vi "UHR-Fleezers Control (host) -TL FB Corrected Ronen semipassive - stepping.vi"(0 "Tab Control":T5(tab)=enum."Trap Control (RF)") -> ()   [LabVIEW 2013] (continued)
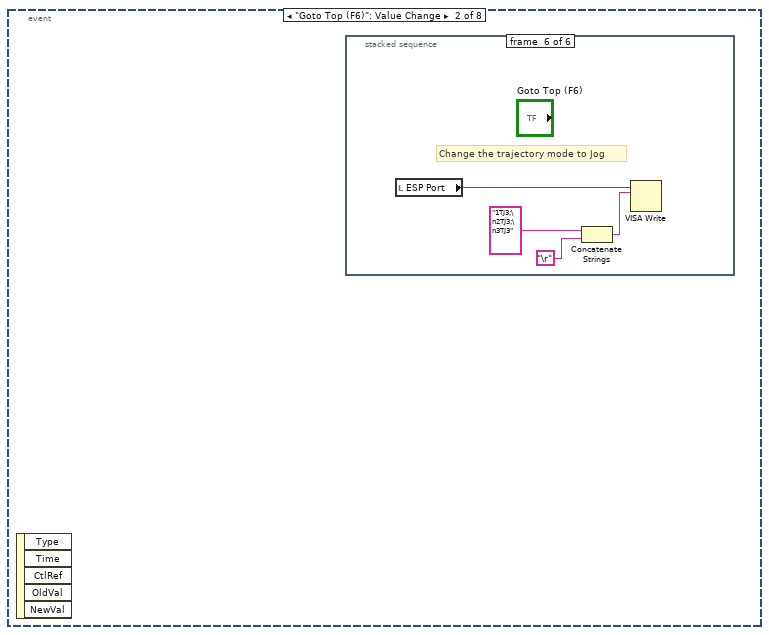
[diagram p4: hidden frame]
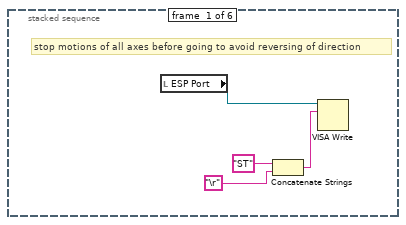
[diagram p5: hidden frame]
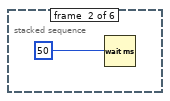
[diagram p6: hidden frame]
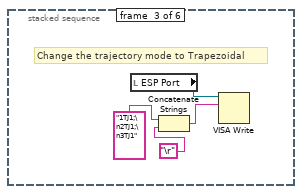
[diagram p7: hidden frame]
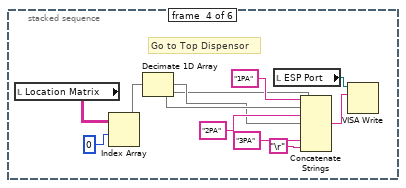
[diagram p8: hidden frame]
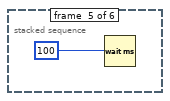
[diagram p9: hidden frame]
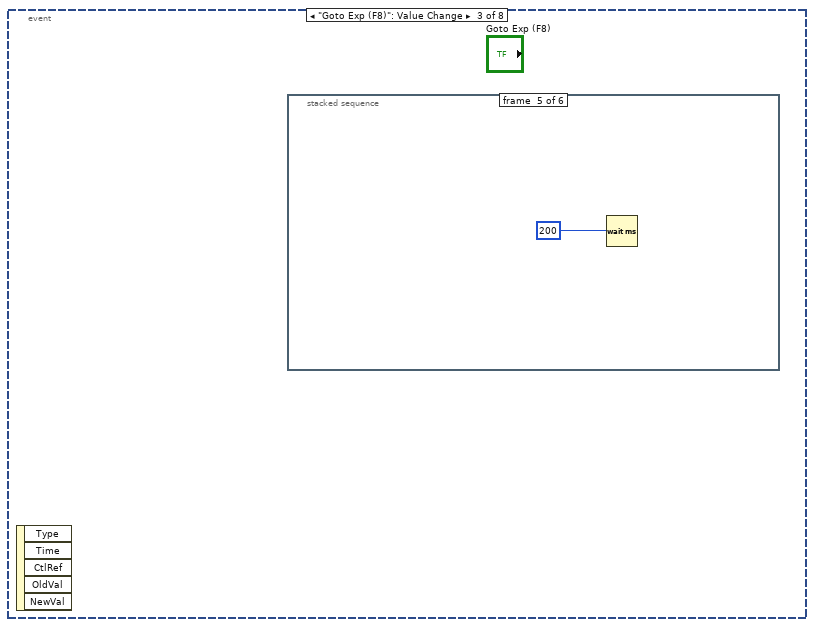
[diagram p10: hidden frame]
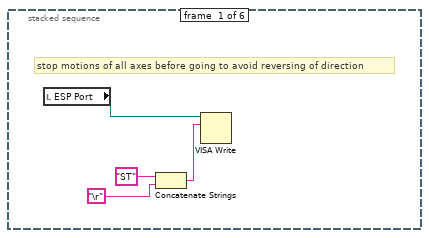
[diagram p11: hidden frame]
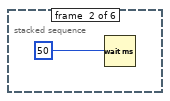
[diagram p12: hidden frame]
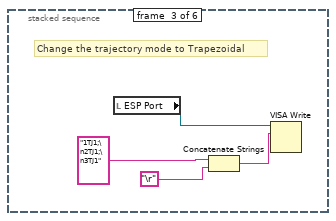
[diagram p13: hidden frame]
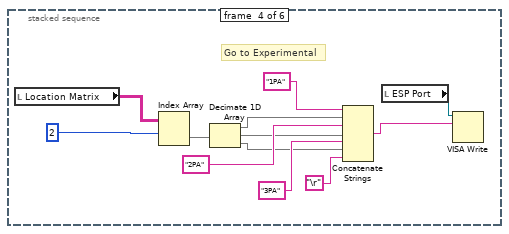
[diagram p14: hidden frame]
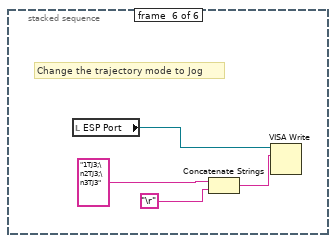
[diagram p15: hidden frame]
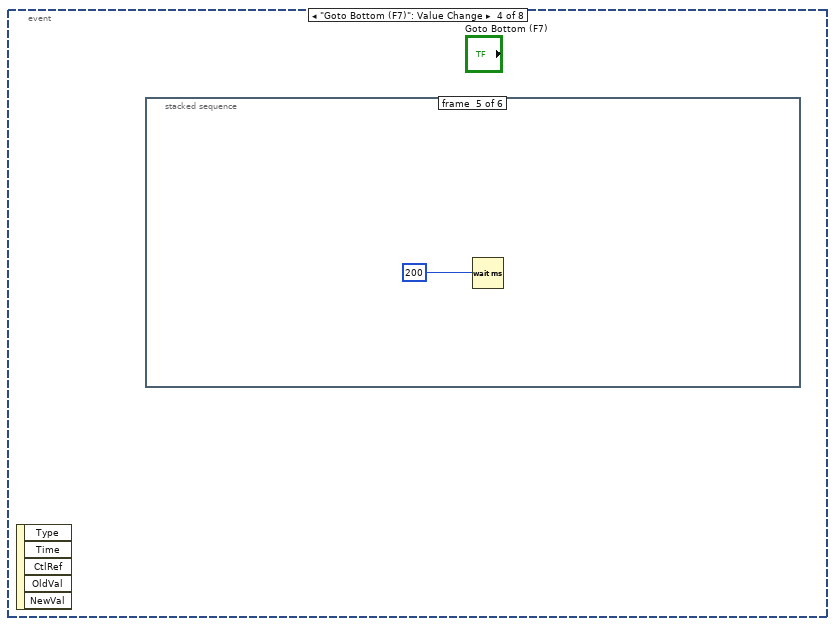
[diagram p16: hidden frame]
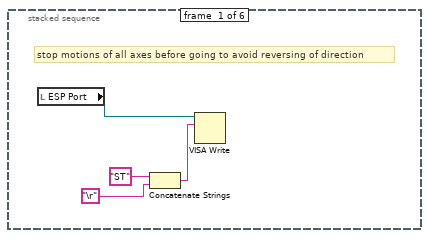
[diagram p17: hidden frame]
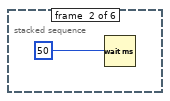
[diagram p18: hidden frame]
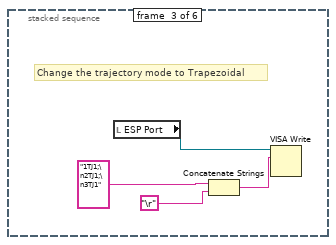
[diagram p19: hidden frame]
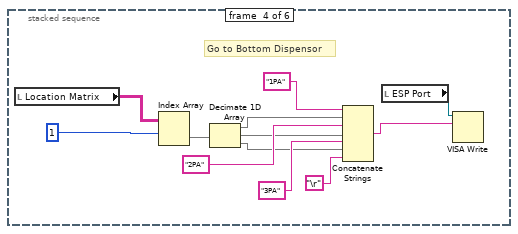
[diagram p20: hidden frame]
                n2311 = call-poly <vilib>:"Mean.vi"("X"=w3787) -> ("mean"=w3780:dbl)  [unwired: 1 out]
                n2312 = Subtract(x=w3781, y=w3780) -> (x-y=w3771:dbl)
                "Delta Fl. 2" <- w3771
                n2313 = Subtract(x=w3806, y=w3805) -> (x-y=w3803:dbl)
                "Delta Fl. 1" <- w3803
                n2314 = Initialize Array(w3803, 1 ("dimension size")) -> (w3800:dbl[])
                n2315 = Initialize Array(w3771, 1 ("dimension size")) -> (w3777:dbl[])
                n2316 = feedback #29(w3800) -> (w3801:dbl[])
                n2317 = Build Array (concatenate)(w3801, w3800) -> (w3799:dbl[])
                n2318 = feedback #30(w3777) -> (w3778:dbl[])
                n2319 = Build Array (concatenate)(w3778, w3777) -> (w3776:dbl[])
                n2320 = Select(t=w3800, s=w3772, f=w3799) -> (s? t:f=w3775:dbl[])
                n2321 = feedback-in #29(w3775) -> ()
                n2322 = Select(t=w3777, s=w3772, f=w3776) -> (s? t:f=w3774:dbl[])
                n2323 = feedback-in #30(w3774) -> ()
                n2324 = Build Array(w3775, w3774) -> (→"Save APD Deriv":dbl[][])
              }
            }
            "Progress" <- w3748
            "Progress 2" <- w3748
          }
        }
      }
    }
    n2325 = Bundle By Name(cluster=w2398, "Green FB Ch 0"=w2397, "Green FB Ch 1"=w2396) -> (w2380:T49)
    "Green FB Signals (V)" <- w2380
    n2326 = Unbundle By Name(w2380) -> ("Green FB Ch 2"=→"Green FB Plot":dbl)
    n2327 = local read "wait to reset values"() -> (w2466:bool)
    n2328 = Not(x=w2463) -> (.not. x?=w2467:bool)
    n2329 = And(x=w2467, y=w2466) -> (x .and. y?=w2468:bool)
    n2330 = case "Part of MCL raster scanning: returns to initial positions after scan done" shown="False" w2468 {
      tunnel: w2471 -> [w3300 w3307]
      tunnel: [w3300 w3306] -> w2470
      tunnel: w2465 -> [w3299 w3305]
      tunnel: [w3299 w3304] -> w2464
      frame False {
      }
      frame True {
        w3315 = 10.0 ("y")
        w3314 = 32767.0 ("y")
        # "to return scan values\nafter a synchronous \nAOM scan"
        n2331 = local read "AO2"() -> (w3308:dbl)
        n2332 = local read "AO1"() -> (w3309:dbl)
        n2333 = local write "wait to reset values"(FALSE ("wait to reset values")) -> ()
        n2334 = Multiply(x=w3309, y=w3314) -> (x*y=w3311:dbl)
        n2335 = Multiply(x=w3308, y=w3314) -> (x*y=w3313:dbl)
        n2336 = Divide(x=w3311, y=w3315) -> (x/y=w3310:dbl)
        n2337 = Divide(x=w3313, y=w3315) -> (x/y=w3312:dbl)
        n2338 = To Word Integer(number=w3310) -> (16bit integer=w3316:i16)
        n2339 = To Word Integer(number=w3312) -> (16bit integer=w3317:i16)
        n2340 = local read "Total Counts (ticks)"() -> (w3301:u32)
        n2341 = xnode "Read/Write Control"("FPGA VI Reference In"=w3307, "error in"=w3305, "AO1"=w3316, "AO2"=w3317, "MCL count"=w3301) -> ("FPGA VI Reference Out"=w3306:T20, "error out"=w3304:errorcluster)
        n2342 = local read "Scan Range (V)\n(of steps)"() -> (w3302:dbl)
        n2343 = property on="Scan Range (V)\n(of steps)" class="DigNum (strict)"("Val(Sgnl)"=w3302) -> ()  [unwired: 2 in, 2 out]
      }
    }
    n2344 = node-c288() -> ()  [unwired: 2 out]
  }
  n2345 = node-c288(3 ("Processor")) -> (w94:T25)  [unwired: 3 out]
  n2346 = timed-loop "Oscillate AOD (debugging)" {
    tunnel: w44 -> [w3876]
    tunnel: [w3875] -> w56
    timing: w94 -> [_]
    timing-out: [_] -> w93
    stop <- w3875 stop-if-true
    n2347 = node-c288() -> ()  [unwired: 2 out]
    n2348 = event shown="[0] \"Oscillate Set 2\", \"Fish for Tether\": Value Change" {
      selector: _ -> [_ _ _]
      dyn-events: _ -> [_ _ _]
      timeout: _ -> [_ _ _]
      tunnel: w3876 -> [w3883 _ _]
      tunnel: [FALSE ("Stop All") _ w4151] -> w3875
      event "Oscillate Set 2", "Fish for Tether": Value Change {
        n2349 = event-data() -> ()  [unwired: 6 out]
        n2350 = local read "Oscillate Set 2"() -> (w3882:bool)
        n2351 = Or(x=w3882, y="Fish for Tether") -> (x .or. y?=w3880:bool)
        n2352 = case shown="True" w3880 {
          tunnel: w3883 -> [_ w3886]
          tunnel: "Fish for Tether" -> [_ w3885]
          frame False {
          }
          frame True {
            n2353 = case shown="True" w3885 {
              frame False {
              }
              frame True {
                n2354 = local write "Scan axis 2"(TRUE) -> ()
                n2355 = local write "Tether"(FALSE ("Tether")) -> ()
              }
            }
            n2356 = node-c288("Period") -> (w3888:T25)  [unwired: 3 out]
            n2357 = timed-loop "Oscillate AOD" {
              timing: w3888 -> [_]
              timing-out: [_] -> w3887
              tunnel: w3886 -> [w3898]
              tunnel: w3885 -> [w3897]
              i -> [w3900]
              stop <- w3896 stop-if-true
              n2358 = node-c288() -> (w3899:i64)  [unwired: 1 out]
              n2359 = flat-sequence {
                tunnel: w3900 -> [w3926]
                tunnel: w3899 -> [w3925]
                tunnel: w3898 -> [w3909]
                tunnel: w3897 -> [w3911]
                tunnel: [w3911] -> w3895
                tunnel: [w3910] -> w3894
                tunnel: [w3908] -> w3893
                tunnel: [w3905] -> w3891
                tunnel: w3895 -> [w3962]
                tunnel: w3894 -> [w3960]
                tunnel: w3893 -> [w3959]
                tunnel: [w3958] -> w3892
                tunnel: w3891 -> [w3957]
                tunnel: [w4026] -> w3896
                tunnel: w3892 -> [w4024]
                frame #0 {
                  n2360 = Divide(x=w3925, y=i64 1000) -> (x/y=w3920:dbl)
                  n2361 = Multiply(x=w3920, y=w3926) -> (x*y=w3922:dbl)
                  n2362 = Multiply(x="Osc. freq. (Hz)", y=6.283185307179586) -> (x*y=w3923:dbl)
                  n2363 = Multiply(x=w3923, y=w3922) -> (x*y=w3907:dbl)
                  n2364 = local read "BD 1 Frequency 2 (MHz)"() -> (w3904:dbl)
                  n2365 = local read "BD 1 Frequency 1 (MHz)"() -> (w3901:dbl)
                  n2366 = case shown="True" w3911 {
                    tunnel: w3907 -> [w3932 w3939]
                    tunnel: w3904 -> [_ w3949]
                    tunnel: [w3929 w3933] -> w3912
                    tunnel: [FALSE w3942] -> w3908
                    tunnel: [0.0 w3935] -> w3905
                    tunnel: w3901 -> [_ w3934]
                    frame False {
                      n2367 = Sine(x=w3932) -> (sin(x)=w3930:dbl)
                      n2368 = Multiply(x=w3930, y="Osc. amp. (MHz)") -> (x*y=w3929:dbl)
                    }
                    frame True {
                      n2369 = Cosine(x=w3939) -> (cos(x)=w3952:dbl)
                      n2370 = Subtract(x=w3949, y=w3934) -> (x-y=w3948:dbl)
                      n2371 = Decrement(x=w3952) -> (x-1=w3951:dbl)
                      n2372 = Subtract(x=w3948, y="Closest Delta (MHz)") -> (x-y=w3945:dbl)
                      n2373 = Divide(x=w3951, y=2.0) -> (x/y=w3946:dbl)
                      n2374 = Multiply(x=w3946, y=w3945) -> (x*y=w3933:dbl)
                      n2375 = local read "Vec Mean of T1 T2"() -> (w3941:dbl[])
                      n2376 = Greater?(x=w3941, y="Stop F (pN)") -> (0:w3943:bool[])
                      n2377 = Or Array Elements(Boolean array=w3943) -> (logical OR=w3942:bool)
                      n2378 = Divide(x=w3939, y=6.283185307179586) -> (x/y=w3938:dbl)
                      n2379 = Round Toward +Infinity(x=w3938) -> (ceil(x): smallest int >= x=w3935:dbl)
                      "Attempts" <- w3935
                      n2380 = Greater?(x=w3935, y="Attempt Limit") -> (0:w3937:bool)
                      n2381 = case shown="True" w3937 {
                        frame False {
                        }
                        frame True {
                          n2382 = local write "Fish for Tether"(FALSE ("Fish for Tether")) -> ()
                          n2383 = call <vilib>:"Beep.vi"() -> ()  [unwired: 3 in, 9 out]
                          n2384 = local read "Messages"() -> (w3954:string)
                          n2385 = call "Update messages.vi"("Message to add"="Tether fishing timeout." ("Messages"), "Old message string"=w3954) -> ("New message string"=→"Messages":string)
                        }
                      }
                    }
                  }
                  n2386 = local read "Y RF Frequency Limits (MHz)"() -> (w3913:T17)
                  n2387 = local read "X RF Frequency Limits (MHz)"() -> (w3914:T17)
                  n2388 = local read "BD 1 Frequency 3 (MHz)"() -> (w3919:dbl)
                  n2389 = local read "BD 2 Frequency 2 (MHz)"() -> (w3903:dbl)
                  n2390 = Select(t=w3904, s="Scan axis 2", f=w3903) -> (s? t:f=w3915:dbl)
                  n2391 = Add(x=w3912, y=w3915) -> (x+y=w3910:dbl)
                  n2392 = Select(t=w3910, s="Scan axis 2", f=w3904) -> (s? t:f=w3902:dbl)
                  n2393 = Select(t=w3903, s="Scan axis 2", f=w3910) -> (s? t:f=w3917:dbl)
                  n2394 = local read "BD 2 Frequency 3 (MHz)"() -> (w3918:dbl)
                  n2395 = call "set RF board frequency - interlace.vi"("Board 2 Frequency Limits"=w3913, "Board 1 Frequency Limits"=w3914, "FPGA VI Reference In"=w3909, "Board 2 Frequency 3 (MHz)"=w3918, "Board 1 Frequency 3 (MHz)"=w3919, "Board 2 Frequency 2 (MHz)"=w3903, "Board 2 Frequency 1 (MHz)"=w3917, "Board 1 Frequency 2 (MHz)"=w3902, "Board 1 Frequency 1  (MHz)"=w3901) -> ()  [unwired: 1 in, 2 out]
                }
                frame #1 {
                  n2396 = And(x=w3962, y=w3959) -> (x .and. y?=w3961:bool)
                  n2397 = case "Only if were fishing and now formed tether" shown="True" w3961 {
                    tunnel: w3960 -> [w3964 w3976]
                    tunnel: [w3963 w3975] -> w3958
                    tunnel: w3957 -> [_ w3971]
                    frame False {
                      n2398 = local read "Fish for Tether"() -> (w3963:bool)
                      n2399 = case shown="True" w3963 {
                        tunnel: w3964 -> [_ _]
                        frame False {
                        }
                        frame True {
                        }
                      }
                    }
                    frame True {
                      w3975 = FALSE ("Fish for Tether")
                      n2400 = call <vilib>:"Beep.vi"() -> ()  [unwired: 3 in, 9 out]
                      n2401 = Number To Decimal String(number=w3971, width (-)=i16 1) -> (decimal integer string=w3969:string)
                      n2402 = case shown="\"2\", \"3\", \"4\", \"5\", \"6\"" "Then..." {
                        selector: "Then..." -> [_ w3979]
                        tunnel: w3976 -> [w3978 _]
                        frame "1", Default {
                          # "do nothing"
                          n2403 = property on="BD 1 Frequency 1 (MHz)" class="DigNum (strict)"("Val(Sgnl)"=w3978) -> ()  [unwired: 2 in, 2 out]
                        }
                        frame "2", "3", "4", "5", "6" {
                          n2404 = flat-sequence {
                            tunnel: w3979 -> [w3981]
                            frame #0 {
                              n2405 = property on="Trap Delta (MHz)" class="DigNum (strict)"("Val(Sgnl)"="Move to Delta 1 (MHz)") -> ()  [unwired: 2 in, 2 out]
                            }
                            frame #1 {
                              n2406 = case shown="\"5\", \"6\"" w3981 {
                                selector: w3981 -> [w3984 w3994 _]
                                frame "3", "4" {
                                n2407 = flat-sequence {
                                tunnel: w3984 -> [w3985]
                                tunnel: [w3985] -> w3982
                                tunnel: [w3987] -> w3983
                                tunnel: w3982 -> [w3987]
                                tunnel: w3983 -> [w3991]
                                frame #0 {
                                n2408 = property on="Green Laser ON/Interlacing" class="Bool (strict)"("Val(Sgnl)"=TRUE ("Value (Signaling)")) -> ()  [unwired: 2 in, 2 out]
                                }
                                frame #1 {
                                n2409 = Multiply(x="Wait Before Save (s)", y=u32 1000 ("x")) -> (x*y=w3989:u32)
                                n2410 = Wait (ms)(milliseconds to wait=w3989) -> ()  [unwired: 1 out]
                                }
                                frame #2 {
                                n2411 = property on="Start Saving" class="Bool (strict)"("Value"=TRUE ("Start Saving")) -> ()  [unwired: 2 in, 2 out]
                                n2412 = case shown="Default" w3991 {
                                frame Default {
                                }
                                frame "4" {
                                n2413 = property on="Fl. Triggered..." class="Bool (strict)"("Val(Sgnl)"=TRUE ("Value (Signaling)")) -> ()  [unwired: 2 in, 2 out]
                                }
                                }
                                }
                                }
                                }
                                frame "5", "6" {
                                n2414 = stacked-sequence {
                                tunnel: w3994 -> [_ _ _ _ _ _ _ _ w4011 _ _]
                                frame #0 {
                                n2415 = Replace Array Subset(array=u32[] [0] ("Index Values"), new element="Raster Set Upon Tether", index=0) -> (w3995:u32[])
                                n2416 = property on="Saved AOD Raster Scan Parameter Sets" class="Arr (strict)"("Index Values"=w3995) -> ()  [unwired: 2 in, 2 out]
                                }
                                frame #1 {
                                n2417 = Wait (ms)(milliseconds to wait=u32 500) -> ()  [unwired: 1 out]
                                }
                                frame #2 {
                                n2418 = property on="Load parameters" class="Bool (strict)"("Val(Sgnl)"=TRUE ("Value (Signaling)")) -> ()  [unwired: 2 in, 2 out]
                                }
                                frame #3 {
                                n2419 = Wait (ms)(milliseconds to wait=u32 500) -> ()  [unwired: 1 out]
                                }
                                frame #4 {
                                n2420 = property on="Trap Raster Scan" class="Bool (strict)"("Val(Sgnl)"=TRUE ("Value (Signaling)")) -> ()  [unwired: 2 in, 2 out]
                                }
                                frame #5 {
                                n2421 = Wait (ms)(milliseconds to wait=u32 2000) -> ()  [unwired: 1 out]
                                }
                                frame #6 {
                                n2422 = while {
                                stop <- w4006 stop-if-true
                                n2423 = local read "Raster Scanning..."() -> (w4005:bool)
                                n2424 = local read "Saving..."() -> (w4008:bool)
                                n2425 = Wait (ms)(milliseconds to wait=u32 100) -> ()  [unwired: 1 out]
                                n2426 = Not(x=w4008) -> (.not. x?=w4007:bool)
                                n2427 = Not(x=w4005) -> (.not. x?=w4004:bool)
                                n2428 = And(x=w4007, y=w4004) -> (x .and. y?=w4006:bool)
                                }
                                }
                                frame #7 {
                                n2429 = property on="Trap Delta (MHz)" class="DigNum (strict)"("Val(Sgnl)"="Move to Delta 2 (MHz)") -> ()  [unwired: 2 in, 2 out]
                                }
                                frame #8 {
                                n2430 = local read "Tether"() -> (w4012:bool)
                                n2431 = case shown="True" w4012 {
                                tunnel: w4011 -> [_ w4013]
                                frame False {
                                }
                                frame True {
                                n2432 = flat-sequence {
                                tunnel: w4013 -> [w4015]
                                frame #0 {
                                n2433 = Wait (ms)(milliseconds to wait=u32 500) -> ()  [unwired: 1 out]
                                }
                                frame #1 {
                                n2434 = case shown="\"6\"" w4015 {
                                frame Default {
                                }
                                frame "6" {
                                n2435 = property on="Green Laser ON/Interlacing" class="Bool (strict)"("Val(Sgnl)"=TRUE ("Green Laser ON/Interlacing")) -> ()  [unwired: 2 in, 2 out]
                                }
                                }
                                }
                                frame #2 {
                                n2436 = Wait (ms)(milliseconds to wait=u32 500) -> ()  [unwired: 1 out]
                                }
                                frame #3 {
                                n2437 = local write "Start Saving"("Save at end (5, 6)") -> ()
                                }
                                }
                                }
                                }
                                }
                                frame #9 {
                                n2438 = local read "Bead Sep. Int. Time (s)"() -> (w4021:dbl)
                                n2439 = Multiply(x=w4021, y=1000.0) -> (x*y=w4020:dbl)
                                n2440 = Wait (ms)(milliseconds to wait=w4020) -> ()  [unwired: 1 out]
                                }
                                frame #10 {
                                n2441 = property on="Rescale on Mean" class="Bool (strict)"("Val(Sgnl)"=TRUE ("Value (Signaling)")) -> ()  [unwired: 2 in, 2 out]
                                }
                                }
                                }
                                frame "2", Default {
                                }
                              }
                            }
                          }
                        }
                      }
                      n2442 = Concatenate Strings("Formed tether in ", w3969, " attempt(s)." ("string")) -> (w3966:string)
                      n2443 = local read "Messages"() -> (w3973:string)
                      n2444 = local write "Fish for Tether"(w3975) -> ()
                      n2445 = call "Update messages.vi"("Message to add"=w3966, "Old message string"=w3973) -> ("New message string"=w3972:string)
                      n2446 = local write "Messages"(w3972) -> ()
                      n2447 = Get Date/Time In Seconds() -> (seconds since 1Jan1904=→"Time tether formed":timestamp)
                      "Tether" <- "Tether Alarm?"
                    }
                  }
                }
                frame #2 {
                  n2448 = local read "Oscillate Set 2"() -> (w4025:bool)
                  n2449 = local read "Stop All"() -> (w4027:bool)
                  n2450 = Not Or(1:w4024, 2:w4025) -> (0:w4023:bool)
                  n2451 = Compound Arithmetic op=OR(w4027, w4023) -> (w4026:bool)
                }
              }
              n2452 = node-c288() -> ()  [unwired: 2 out]
            }
            n2453 = node-c288(w3887) -> ()  [unwired: 1 out]
          }
        }
      }
      event "Fl. Triggered...": Value Change {
        n2454 = event-data() -> ()  [unwired: 7 out]
        n2455 = case shown="True" "Fl. Triggered..." {
          frame False {
          }
          frame True {
            n2456 = node-c288() -> (w4039:T25)  [unwired: 4 out]
            n2457 = timed-loop {
              timing: w4039 -> [_]
              timing-out: [_] -> w4038
              tunnel: "Action" -> [w4043]
              shift-right: [w4040] -> _
              shift-left: u8 255 -> [w4042]
              stop <- w4044 stop-if-true
              n2458 = node-c288() -> ()  [unwired: 2 out]
              n2459 = flat-sequence {
                tunnel: w4043 -> [w4056]
                tunnel: w4042 -> [w4053]
                tunnel: [w4052] -> w4041
                tunnel: [w4142] -> w4044
                tunnel: w4041 -> [w4141]
                tunnel: [w4141] -> w4040
                frame #0 {
                  n2460 = local read "Delta Fl. 2"() -> (w4047:dbl)
                  n2461 = local read "Delta Fl. 1"() -> (w4048:dbl)
                  n2462 = Select(t=w4048, s="APD to Watch", f=w4047) -> (s? t:f=w4046:dbl)
                  n2463 = Multiply(x="Fl. Delta Thresh. (kHz)", y=1000.0) -> (x*y=w4055:dbl)
                  n2464 = Greater?(x=w4046, y=w4055) -> (0:w4050:bool)
                  n2465 = Or(x="Force Yank", y=w4050) -> (x .or. y?=w4051:bool)
                  n2466 = case shown="True" w4051 {
                    tunnel: w4056 -> [_ w4066]
                    tunnel: w4053 -> [w4058 w4062]
                    tunnel: [w4058 w4059] -> w4052
                    frame False {
                    }
                    frame True {
                      n2467 = flat-sequence {
                        tunnel: w4063 -> [w4072]
                        tunnel: [w4072] -> w4067
                        tunnel: w4066 -> [w4071]
                        tunnel: [w4071] -> w4065
                        tunnel: [w4070] -> w4064
                        tunnel: w4062 -> [w4069]
                        tunnel: [w4068] -> w4061
                        tunnel: w4067 -> [w4097]
                        tunnel: w4065 -> [w4096]
                        tunnel: w4064 -> [w4095]
                        tunnel: w4061 -> [w4094]
                        tunnel: [w4094] -> w4060
                        tunnel: w4060 -> [w4139]
                        tunnel: [w4139] -> w4059
                        frame #0 {
                          n2468 = call <vilib>:"Beep.vi"() -> ()  [unwired: 3 in, 9 out]
                          n2469 = local write "Waiting"(FALSE ("Waiting")) -> ()
                          n2470 = Increment(x=w4069) -> (x+1=w4068:u8)
                          n2471 = case shown="\"Yank\"" w4071 {
                            tunnel: w4068 -> [_ _ w4078]
                            frame "Image" {
                              n2472 = property on="Confocal Image" class="Bool (strict)"("Val(Sgnl)"=TRUE ("Value (Signaling)")) -> ()  [unwired: 2 in, 2 out]
                            }
                            frame "Alarm", Default {
                            }
                            frame "Yank" {
                              n2473 = flat-sequence {
                                tunnel: w4078 -> [w4081]
                                tunnel: [w4080] -> w4077
                                tunnel: ["N Array El"] -> w4076
                                tunnel: w4077 -> [w4091]
                                tunnel: w4076 -> [w4087]
                                frame #0 {
                                n2474 = Multiply(x="Yank Delay (s)", y=1000.0) -> (x*y=w4084:dbl)
                                n2475 = Quotient & Remainder(x=w4081, y="N Array El") -> (x-y*floor(x/y)=w4080:u8)  [unwired: 1 out]
                                n2476 = Wait (ms)(milliseconds to wait=w4084) -> ()  [unwired: 1 out]
                                }
                                frame #1 {
                                n2477 = Random Number (0-1)() -> (number: 0 to 1=w4088:dbl)
                                n2478 = Multiply(x=w4087, y=w4088) -> (x*y=w4086:dbl)
                                n2479 = Round Toward -Infinity(1:w4086) -> (0:w4085:dbl)
                                n2480 = Select(t=w4085, s="Random Choice", f=w4091) -> (s? t:f=w4089:dbl)
                                n2481 = Index Array(array="Yank to Delta Array (MHz)", index=w4089) -> (element=w4092:dbl)
                                n2482 = property on="Trap Delta (MHz)" class="DigNum (strict)"("Val(Sgnl)"=w4092) -> ()  [unwired: 2 in, 2 out]
                                }
                              }
                            }
                          }
                          n2483 = local read "Time (s)"() -> (w4070:dbl)
                          "Fl. High" <- TRUE ("Yanking")
                        }
                        frame #1 {
                          n2484 = node-c288() -> (w4099:T25)  [unwired: 4 out]
                          n2485 = timed-loop {
                            timing: w4099 -> [_]
                            timing-out: [_] -> w4098
                            tunnel: w4097 -> [w4115]
                            tunnel: w4096 -> [w4113]
                            tunnel: w4095 -> [w4112]
                            stop <- w4114 stop-if-true
                            n2486 = node-c288() -> ()  [unwired: 2 out]
                            n2487 = local read "Fl. Delta Thresh. (kHz)"() -> (w4107:dbl)
                            n2488 = local read "Fl. Triggered..."() -> (w4116:bool)
                            n2489 = local read "Delta Fl. 1"() -> (w4103:dbl)
                            n2490 = local read "Delta Fl. 2"() -> (w4101:dbl)
                            n2491 = local read "Stop All"() -> (w4110:bool)
                            n2492 = local read "APD to Watch"() -> (w4102:bool)
                            n2493 = Select(t=w4103, s=w4102, f=w4101) -> (s? t:f=w4100:dbl)
                            n2494 = Not(x=w4116) -> (.not. x?=w4111:bool)
                            n2495 = Multiply(x=w4107, y=1000.0) -> (x*y=w4106:dbl)
                            n2496 = Negate(x=w4106) -> (-x=w4105:dbl)
                            n2497 = Less?(x=w4100, y=w4105) -> (x < y?=w4109:bool)
                            n2498 = Compound Arithmetic op=OR(w4109, w4110, w4111, "Force Reset") -> (w4114:bool)
                            n2499 = case shown="True" w4114 {
                              tunnel: w4115 -> [_ w4127]
                              tunnel: w4113 -> [_ w4126]
                              tunnel: w4112 -> [_ w4124]
                              frame False {
                              }
                              frame True {
                                n2500 = case shown="\"Yank\"" w4126 {
                                tunnel: w4127 -> [_ w4128]
                                frame "Image", Default {
                                }
                                frame "Yank" {
                                n2501 = flat-sequence {
                                tunnel: [w4133] -> w4129
                                tunnel: w4128 -> [w4133]
                                tunnel: w4129 -> [w4134]
                                frame #0 {
                                n2502 = local read "Yank Delay (s)"() -> (w4132:dbl)
                                n2503 = Multiply(x=w4132, y=1000.0) -> (x*y=w4130:dbl)
                                n2504 = Wait (ms)(milliseconds to wait=w4130) -> ()  [unwired: 1 out]
                                }
                                frame #1 {
                                n2505 = property on="Trap Delta (MHz)" class="DigNum (strict)"("Val(Sgnl)"=w4134) -> ()  [unwired: 2 in, 2 out]
                                }
                                }
                                }
                                }
                                n2506 = local read "Time (s)"() -> (w4125:dbl)
                                n2507 = Subtract(x=w4125, y=w4124) -> (x-y=w4121:dbl)
                                "Duration (s)" <- w4121
                                n2508 = Number To Decimal String(number=w4121, width (-)=i16 0) -> (decimal integer string=w4119:string)
                                n2509 = Concatenate Strings(w4119, " s fluorescence event." ("string")) -> (w4117:string)
                                n2510 = local read "Messages"() -> (w4123:string)
                                n2511 = call "Update messages.vi"("Message to add"=w4117, "Old message string"=w4123) -> ("New message string"=w4122:string)
                                n2512 = call <vilib>:"Beep.vi"() -> ()  [unwired: 3 in, 9 out]
                                n2513 = local write "Messages"(w4122) -> ()
                              }
                            }
                            n2514 = node-c288() -> ()  [unwired: 2 out]
                          }
                          n2515 = node-c288(w4098) -> ()  [unwired: 1 out]
                        }
                        frame #2 {
                          n2516 = local write "Fl. High"(FALSE ("Yanking")) -> ()
                        }
                      }
                      n2517 = local read "Trap Delta (MHz)"() -> (w4063:dbl)
                    }
                  }
                }
                frame #1 {
                  n2518 = local read "Stop All"() -> (w4145:bool)
                  n2519 = local read "Fl. Triggered..."() -> (w4143:bool)
                  n2520 = Not(x=w4143) -> (.not. x?=w4144:bool)
                  n2521 = Or(x=w4144, y=w4145) -> (x .or. y?=w4142:bool)
                  n2522 = Not(x=w4142) -> (.not. x?=→"Waiting":bool)
                }
              }
              n2523 = node-c288() -> ()  [unwired: 2 out]
            }
            n2524 = node-c288(w4038) -> ()  [unwired: 1 out]
          }
        }
      }
      event "Stop All": Value Change {
        n2525 = event-data() -> ()  [unwired: 7 out]
        n2526 = local read "Stop All"() -> (w4151:bool)
      }
    }
    n2527 = node-c288() -> ()  [unwired: 2 out]
  }
  n2528 = node-c288(w93) -> ()  [unwired: 1 out]
  n2529 = node-c288(w181) -> ()  [unwired: 1 out]
  n2530 = flat-sequence {
    tunnel: w53 -> [w4156]
    tunnel: [w4155] -> w59
    tunnel: [w4152] -> w58
    tunnel: w57 -> [_]
    tunnel: w56 -> [_]
    tunnel: w55 -> [_]
    tunnel: w54 -> [_]
    tunnel: w52 -> [w4153]
    tunnel: w59 -> [w4159]
    tunnel: w58 -> [w4158]
    frame #0 {
      w4154 = FALSE ("APD to FIFO")
      n2531 = xnode "Read/Write Control"("FPGA VI Reference In"=w4156, "error in"=w4153, "APD to FIFO"=w4154, "AI to FIFO"=w4154) -> ("FPGA VI Reference Out"=w4155:T20, "error out"=w4152:errorcluster)
    }
    frame #1 {
      n2532 = xnode "Invoke Method"("FPGA VI Reference In"=w4159, "error in"=w4158) -> ("FPGA VI Reference Out"=w4157:T20)  [unwired: 1 out]
      n2533 = xnode "Close FPGA VI Reference"("FPGA VI Reference In"=w4157) -> ()  [unwired: 1 in, 1 out]
    }
  }
